vi "Point Slope Calibration.vi"(11 "Error In":errorcluster) -> (4 "Pressure Slope":dbl, 6 "Pressure Intercept":dbl, 8 "Flow Array":dbl[](array[numeric]) format="%_6g", 15 "Error Out":errorcluster)   [LabVIEW 2013]
uses:
  <vilib>/Analysis/baseanly.llb/Mean (DBL).vi
  <vilib>/gmath/NI_Gmath.lvlib
  <vilib>/Analysis/NI_AALBase.lvlib
panel:
  out "Flow Calibration":cluster{"Y":dbl[], "Y":dbl[]}[](graph)
  in  "Pressure Reference":dbl min=0.0 max=20.0 step=1.0
  out "Pressure Voltage":dbl
  out "Flow Voltage":dbl
  in  "Flow Reference":dbl min=0.0 max=30.0 step=6.0
  out "Flow Intercept":dbl
  out "Flow Slope":dbl
  in  "Stop Button HS":bool
  in  "Add Button HS":bool
  out "Pressure Curve":cluster{"Y":dbl[], "Y":dbl[]}[](graph)
  out "Flow Curve":cluster{"Y":dbl[], "Y":dbl[]}[](graph)
  # "1. Connect the compressed air to the end of the pressure regulator.\n2. Connect the \"Before\" tube to the P+ port on the Flow side of the Amplifier.\n3. Connect the \"After\" tube to the P- port on.\n4. Connect the pressure calibrator unit to the P+ port on the Pressure side of the Amplifier.\n6. Record voltages and their corresponding pressures by clicking \"Add Value\"\n7. The slope and intercept will be saved for collection."
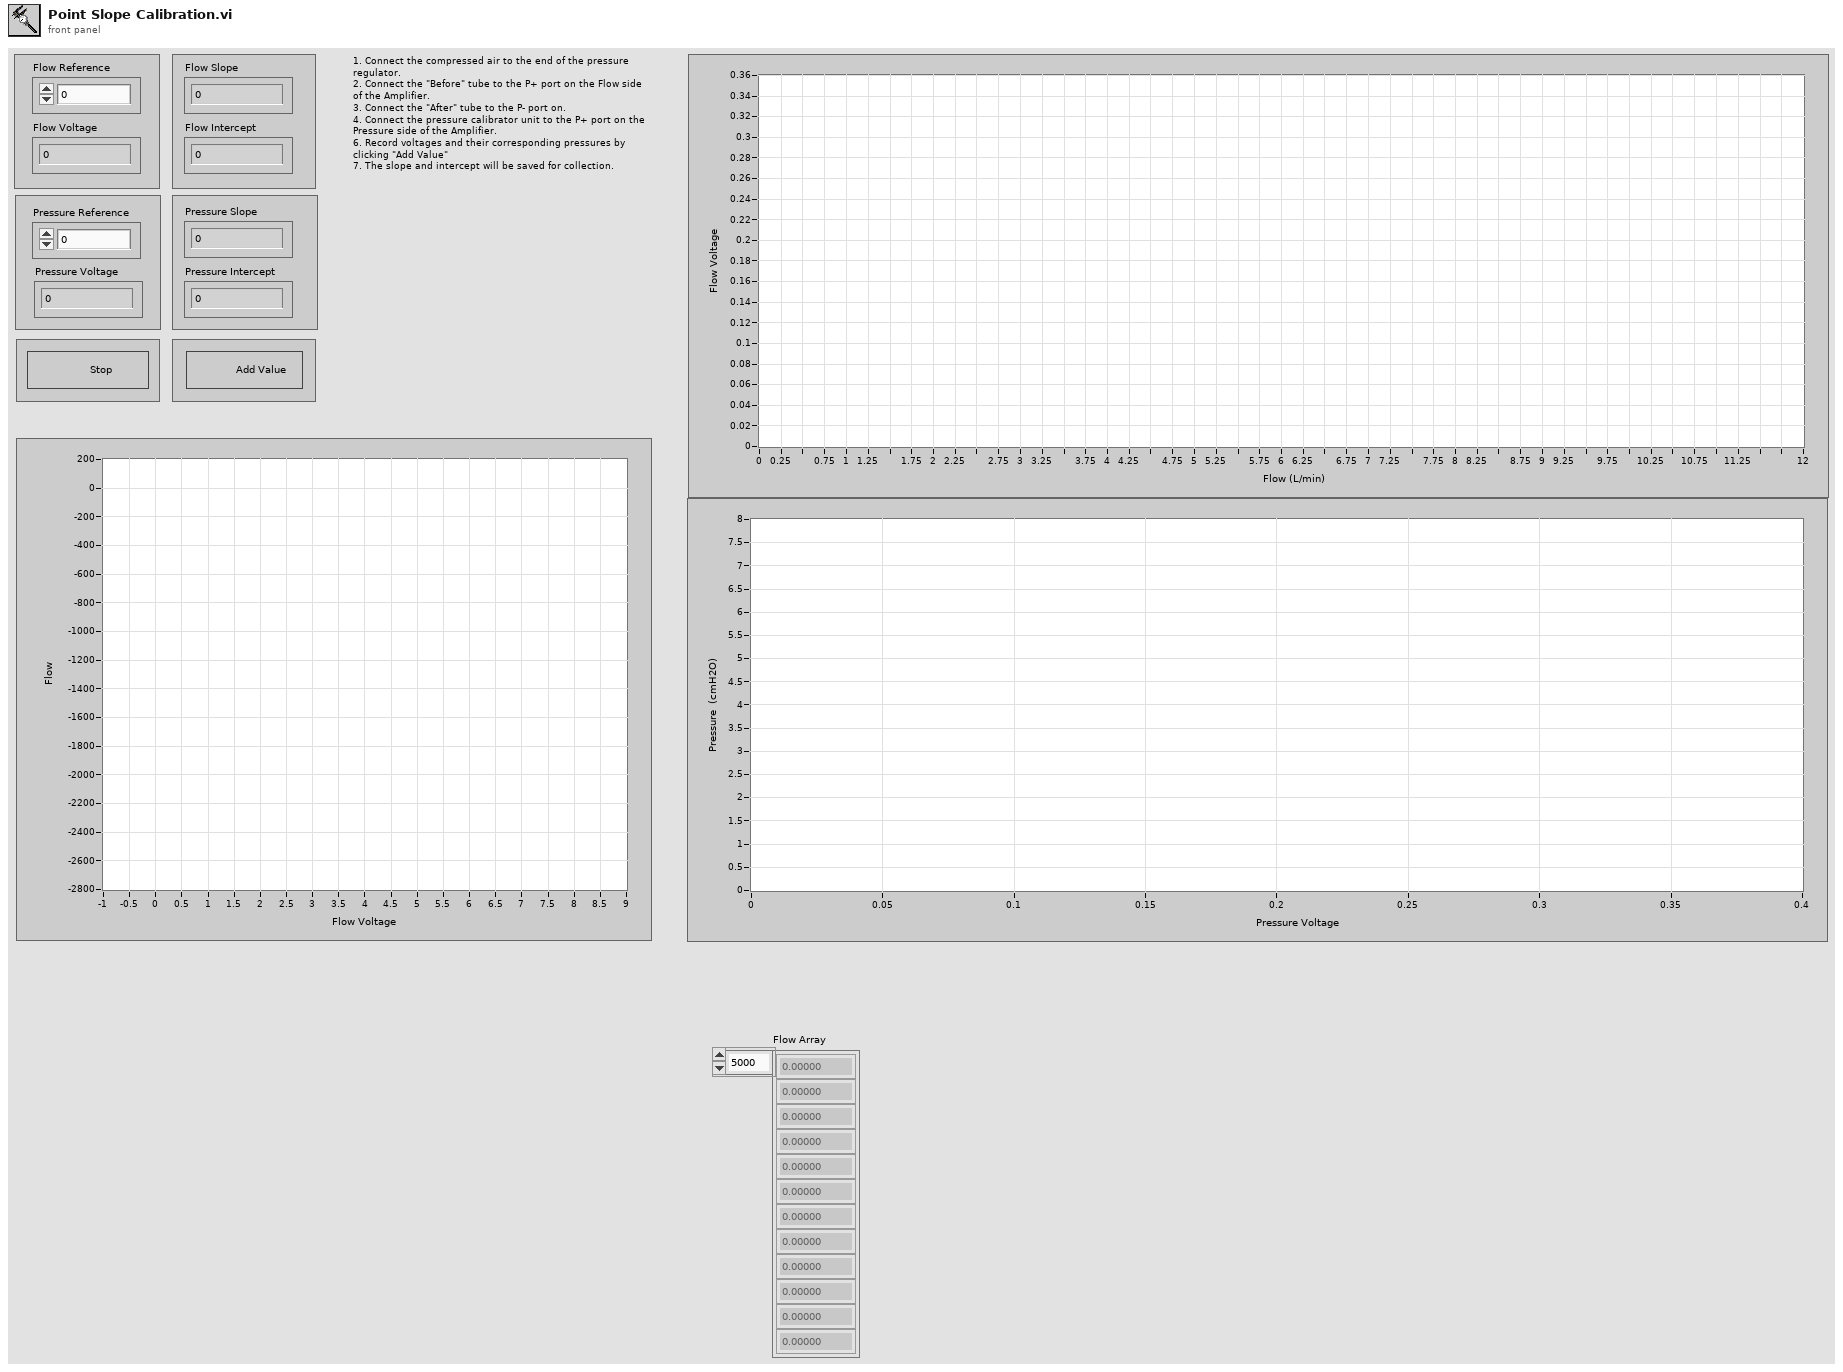
[diagram p1: front panel]
types:
  T1 = enum8{"Enabled", "Disabled", "Disabled and Grayed Out"}
  T2 = cluster{"Volt (Flow)":dbl[], "Ref (Flow)":dbl[]}[]
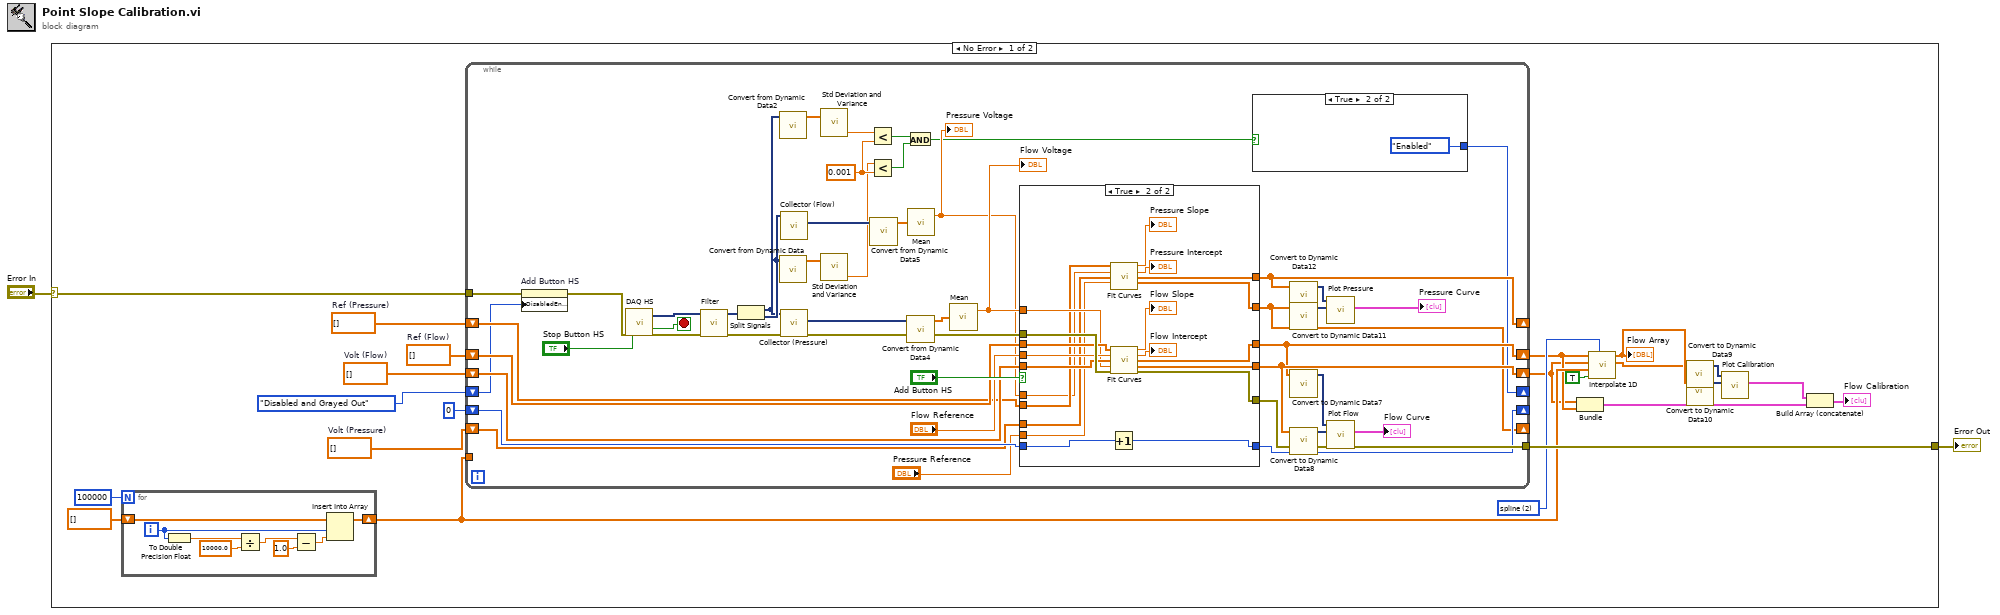
[diagram p0: block diagram]
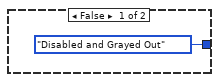
[diagram p2: hidden frame]
diagram:
  n1 = case shown="No Error" "Error In" {
    selector: "Error In" -> [w24 w109]
    tunnel: [w23 w109] -> w1
    frame No Error {
      w6 = dbl[] []  # Ref (Pressure)
      w7 = dbl[] []  # Volt (Pressure)
      w18 = 2 items=["nearest", "linear", "spline", "cubic Hermite", "Lagrange"] ("method")
      w21 = dbl[] []  # Ref (Flow)
      w22 = dbl[] []  # Volt (Flow)
      n2 = for {
        N: 100000 ("dimension size") -> [_]
        shift-right: [w31] -> w12
        shift-left: dbl[] [] -> [w32]
        i -> [w28]
        n3 = To Double Precision Float(number=w28) -> (double precision float=w29:dbl)
        n4 = Divide(x=w29, y=10000.0) -> (x/y=w27:dbl)
        n5 = Subtract(x=w27, y=1.0) -> (x-y=w25:dbl)
        n6 = Insert Into Array(array=w32, index=w28, new element=w25) -> (w31:dbl[])
      }
      n7 = while {
        tunnel: w24 -> [w48]
        shift-right: [w61] -> w4
        shift-left: w22 -> [w63]
        shift-right: [w60] -> w5
        shift-left: w21 -> [w65]
        tunnel: [w68] -> w23
        shift-right: [w66] -> _
        shift-left: 0 -> [w67]
        tunnel: w12 -> [_]
        shift-right: [w53] -> _
        shift-left: w7 -> [w55]
        shift-right: [w54] -> _
        shift-left: w6 -> [w56]
        shift-right: [w40] -> _
        shift-left: T1."Disabled and Grayed Out" ("Disabled") -> [w46]
        stop <- w75 stop-if-true
        w39 = 0.001
        n8 = property on="Add Button HS" class="Bool"(error in=w48, "DisabledEnum"=w46) -> (error out=w47:errorcluster)  [unwired: 1 in, 1 out]
        n9 = call "DAQ HS"("error in"=w47, "stop (F)"="Stop Button HS") -> ("data"=w79:dynamicdata, "stopped"=w75:bool, "error out"=w80:errorcluster)  [unwired: 14 in, 1 out]
        n10 = call "Filter"("error in (no error)"=w80, "Signal"=w79) -> ("error out"=w76:errorcluster, "Filtered Signal"=w58:dynamicdata)  [unwired: 8 in]
        n11 = Split Signals(w58) -> (w33:dynamicdata, w38:dynamicdata)  [unwired: 2 in]
        n12 = call "Convert from Dynamic Data2"("Dynamic Data Type"=w33) -> ("Array"=w37:dbl[])  [unwired: 3 in]
        n13 = call "Convert from Dynamic Data"("Dynamic Data Type"=w38) -> ("Array"=w36:dbl[])  [unwired: 3 in]
        n14 = call "Collector (Flow)"("Signals"=w38) -> ("Collected Signals"=w57:dynamicdata)  [unwired: 9 in, 1 out]
        n15 = call "Collector (Pressure)"("error in (no error)"=w76, "Signals"=w33) -> ("error out"=w72:errorcluster, "Collected Signals"=w74:dynamicdata)  [unwired: 8 in]
        n16 = call <vilib>:"Std Deviation and Variance.vi"("X"=w37) -> ("variance"=w34:dbl)  [unwired: 1 in, 2 out]
        n17 = call <vilib>:"Std Deviation and Variance.vi"("X"=w36) -> ("variance"=w35:dbl)  [unwired: 1 in, 2 out]
        n18 = Less?(x=w34, y=w39) -> (x < y?=w43:bool)
        n19 = Less?(x=w35, y=w39) -> (x < y?=w42:bool)
        n20 = call "Convert from Dynamic Data5"("Dynamic Data Type"=w57) -> ("Array"=w45:dbl[])  [unwired: 3 in]
        n21 = And(x=w43, y=w42) -> (x .and. y?=w41:bool)
        n22 = call "Convert from Dynamic Data4"("Dynamic Data Type"=w74) -> ("Array"=w73:dbl[])  [unwired: 3 in]
        n23 = call-poly <vilib>:"Mean.vi"("X"=w45) -> ("mean"=w44:dbl)  [unwired: 1 out]
        "Pressure Voltage" <- w44
        n24 = call-poly <vilib>:"Mean.vi"("X"=w73) -> ("mean"=w62:dbl)  [unwired: 1 out]
        "Flow Voltage" <- w62
        n25 = case shown="True" "Add Button HS" {
          tunnel: w72 -> [w88 w108]
          tunnel: [w88 w107] -> w71
          tunnel: w67 -> [w87 w106]
          tunnel: [w87 w105] -> w66
          tunnel: w65 -> [w86 w104]
          tunnel: "Flow Reference" -> [_ w103]
          tunnel: w63 -> [w85 w102]
          tunnel: w62 -> [_ w101]
          tunnel: [w86 w100] -> w60
          tunnel: [w85 w99] -> w61
          tunnel: "Pressure Reference" -> [_ w93]
          tunnel: w55 -> [w83 w92]
          tunnel: w56 -> [w84 w94]
          tunnel: w44 -> [_ w91]
          tunnel: [w84 w90] -> w54
          tunnel: [w83 w89] -> w53
          frame False {
          }
          frame True {
            n26 = Increment(x=w106) -> (x+1=w105:i32)
            n27 = call "Fit Curves.vi"("Reference (Array)"=w94, "Reference (Value)"=w91, "Voltage (Array)"=w92, "Voltage (Value)"=w93) -> ("Slope"=→"Pressure Slope":dbl, "Intercept"=→"Pressure Intercept":dbl, "Reference Out"=w90:dbl[], "Voltage Out"=w89:dbl[])  [unwired: 7 in, 1 out]
            n28 = call "Fit Curves.vi"("Reference (Array)"=w104, "Reference (Value)"=w103, "Voltage (Array)"=w102, "Voltage (Value)"=w101, "Error In"=w108) -> ("Slope"=→"Flow Slope":dbl, "Intercept"=→"Flow Intercept":dbl, "Reference Out"=w100:dbl[], "Voltage Out"=w99:dbl[], "Error Out"=w107:errorcluster)  [unwired: 6 in]
          }
        }
        n29 = case shown="True" w41 {
          tunnel: [T1."Disabled and Grayed Out" ("Disabled") T1."Enabled" ("Disabled")] -> w40
          frame False {
          }
          frame True {
          }
        }
        n30 = call "Convert to Dynamic Data12"("Array"=w54) -> ("Dynamic Data Type"=w52:dynamicdata)  [unwired: 3 in]
        n31 = call "Convert to Dynamic Data11"("Array"=w53) -> ("Dynamic Data Type"=w51:dynamicdata)  [unwired: 3 in]
        n32 = call "Convert to Dynamic Data7"("Array"=w60) -> ("Dynamic Data Type"=w69:dynamicdata)  [unwired: 3 in]
        n33 = call "Convert to Dynamic Data8"("Array"=w61) -> ("Dynamic Data Type"=w70:dynamicdata)  [unwired: 3 in]
        n34 = call "Plot Pressure"("Y Input"=w51, "X Input"=w52) -> ("XY Graph"=→"Pressure Curve":cluster{"Y":dbl[], "Y":dbl[]}[])  [unwired: 8 in, 1 out]
        n35 = call "Plot Flow"("error in (no error)"=w71, "Y Input"=w70, "X Input"=w69) -> ("error out"=w68:errorcluster, "XY Graph"=→"Flow Curve":cluster{"Y":dbl[], "Y":dbl[]}[])  [unwired: 7 in]
      }
      n36 = Bundle("Volt (Flow)"=w4, "Ref (Flow)"=w5) -> (w14:cluster{"Volt (Flow)":dbl[], "Ref (Flow)":dbl[]})  [unwired: 1 in]
      n37 = call <vilib>:"Interpolate 1D.vi"("method"=w18, "X is monotonic"=TRUE, "xi"=w12, "X"=w4, "Y"=w5) -> ("xi used"=w9:dbl[], "yi"=w10:dbl[])  [unwired: 4 in, 1 out]
      "Flow Array" <- w10
      n38 = call "Convert to Dynamic Data9"("Array"=w9) -> ("Dynamic Data Type"=w17:dynamicdata)  [unwired: 3 in]
      n39 = call "Convert to Dynamic Data10"("Array"=w10) -> ("Dynamic Data Type"=w16:dynamicdata)  [unwired: 3 in]
      n40 = call "Plot Calibration"("Y Input"=w16, "X Input"=w17) -> ("XY Graph"=w15:cluster{"Y":dbl[], "Y":dbl[]}[])  [unwired: 8 in, 1 out]
      n41 = Build Array (concatenate)(w15, w14) -> (→"Flow Calibration":T2)
    }
    frame Error {
    }
  }
  "Error Out" <- w1
